vi "Check Packets.vi"(1 "A":string, 2 "B":string) -> (0 "A < B?":bool)   [LabVIEW 2022 SP3, in "AoC22.lvlib"]
uses:
  AoC22.lvlib
  Packet Parser.ctl
  Packet Token.ctl
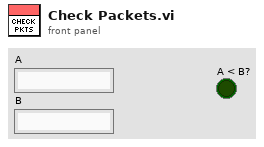
[diagram p1: front panel]
types:
  T1 = typedef "AoC22.lvlib/Packet Parser.ctl" = cluster{"String":string, "Next":i32}
  T2 = typedef "AoC22.lvlib/Packet Token.ctl" = enum16{"List", "End List", "Value", "Comma"}
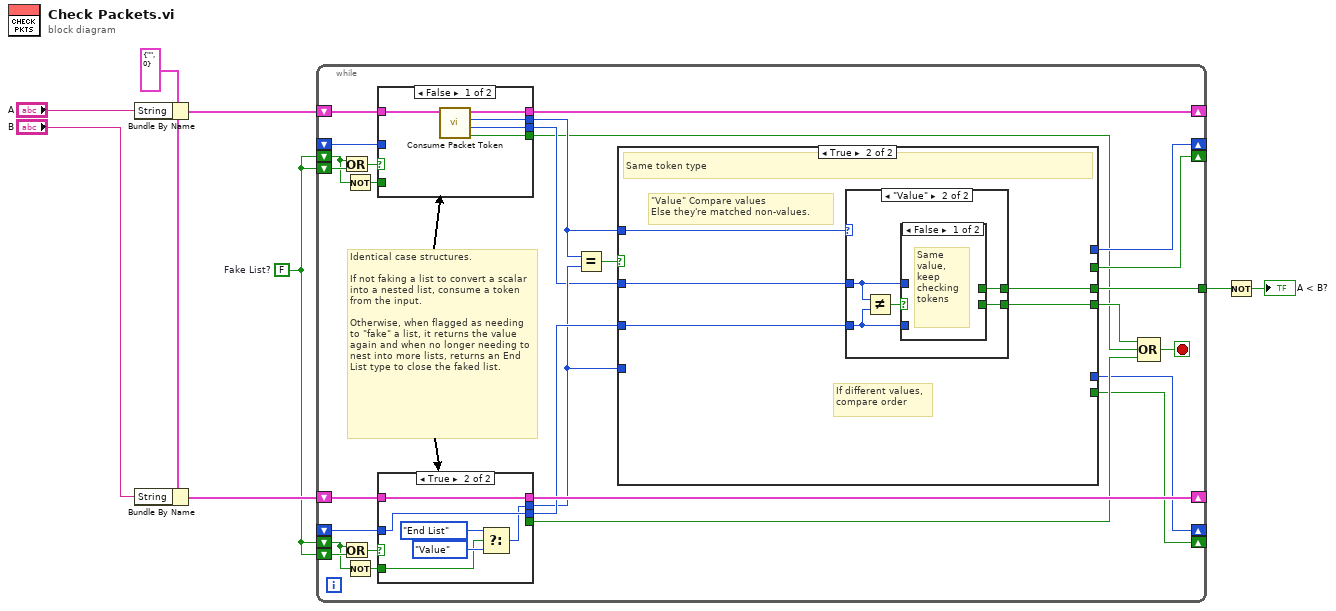
[diagram p0: block diagram]
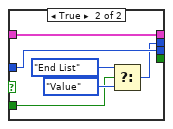
[diagram p2: hidden frame]
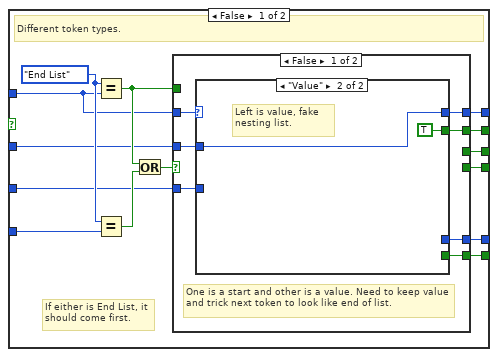
[diagram p3: hidden frame]
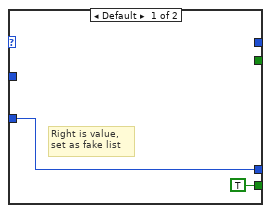
[diagram p4: hidden frame]
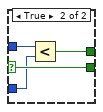
[diagram p7: hidden frame]
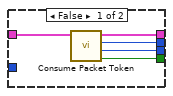
[diagram p8: hidden frame]
diagram:
  w5 = FALSE  # Fake List?
  w8 = T1 {"String"="", "Next"=0} ("Packet Parser")
  n1 = Bundle By Name(cluster=w8, "String"="A") -> (w7:T1)
  n2 = Bundle By Name(cluster=w8, "String"="B") -> (w6:T1)
  n3 = while {
    shift-right: [w16] -> _
    shift-left: w7 -> [w20]
    shift-right: [w34] -> _
    shift-left: w6 -> [w36]
    shift-right: [w25] -> _
    shift-left: w5 -> [w9]
    shift-right: [w24] -> _
    shift-left: w5 -> [w10]
    shift-right: [w26] -> _
    shift-left: _ -> [w19]
    shift-right: [w23] -> _
    shift-left: _ -> [w35]
    tunnel: [w28] -> w4
    shift-left: w5 -> [w17]
    shift-left: w5 -> [w21]
    stop <- w32 stop-if-true
    # "Identical case structures.\n\nIf not faking a list to convert a scalar into a nested list, consume a token from the input.\n\nOtherwise, when flagged as needing to \"fake\" a list, it returns the value again and when no longer needing to nest into more lists, returns an End List type to close the faked list."
    n4 = Or(x=w9, y=w17) -> (x .or. y?=w18:bool)
    n5 = Or(x=w10, y=w21) -> (x .or. y?=w22:bool)
    n6 = Not(x=w9) -> (.not. x?=w12:bool)
    n7 = Not(x=w10) -> (.not. x?=w11:bool)
    n8 = case shown="False" w18 {
      tunnel: w20 -> [w41 w47]
      tunnel: [w40 w47] -> w16
      tunnel: [w39 _] -> w13
      tunnel: [w38 w46] -> w14
      tunnel: [w37 w42] -> w15
      tunnel: w19 -> [_ w46]
      tunnel: w12 -> [_ w43]
      frame False {
        n9 = call "Consume Packet Token.vi"("Packet Parser In"=w41) -> ("End?"=w39:bool, "Value"=w38:i32, "Type"=w37:T2, "Packet Parser"=w40:T1)  [unwired: 7 in]
      }
      frame True {
        n10 = Select(t=Packet_Token."End List" ("Packet Token"), s=w43, f=Packet_Token."Value" ("Packet Token")) -> (s? t:f=w42:T2)
      }
    }
    n11 = case shown="True" w22 {
      tunnel: w36 -> [w93 w99]
      tunnel: [w92 w99] -> w34
      tunnel: [w91 _] -> w33
      tunnel: [w90 w98] -> w30
      tunnel: [w89 w94] -> w27
      tunnel: w35 -> [_ w98]
      tunnel: w11 -> [_ w95]
      frame False {
        n12 = call "Consume Packet Token.vi"("Packet Parser In"=w93) -> ("End?"=w91:bool, "Value"=w90:i32, "Type"=w89:T2, "Packet Parser"=w92:T1)  [unwired: 7 in]
      }
      frame True {
        n13 = Select(t=Packet_Token."End List" ("Packet Token"), s=w95, f=Packet_Token."Value" ("Packet Token")) -> (s? t:f=w94:T2)
      }
    }
    n14 = Equal?(x=w15, y=w27) -> (x = y?=w31:bool)
    n15 = case shown="True" w31 {
      tunnel: w15 -> [w52 w79]
      tunnel: w14 -> [w55 w78]
      tunnel: w30 -> [w54 w77]
      tunnel: [w56 w76] -> w29
      tunnel: [w57 w75] -> w28
      tunnel: w27 -> [w61 _]
      tunnel: [w51 _] -> w26
      tunnel: [w50 _] -> w25
      tunnel: [w49 _] -> w24
      tunnel: [w48 _] -> w23
      frame False {
        w60 = Packet_Token."End List" ("x")
        # "If either is End List, it should come first."
        # "Different token types."
        n16 = Equal?(x=w60, y=w52) -> (x = y?=w58:bool)
        n17 = Equal?(x=w60, y=w61) -> (x = y?=w59:bool)
        n18 = Or(x=w58, y=w59) -> (x .or. y?=w53:bool)
        n19 = case shown="False" w53 {
          selector: w53 -> [_ w73]
          tunnel: w58 -> [_ w74]
          tunnel: [_ w74] -> w57
          tunnel: [_ w73] -> w56
          tunnel: w55 -> [w67 _]
          tunnel: w54 -> [w64 _]
          tunnel: w52 -> [w68 _]
          tunnel: [w66 _] -> w51
          tunnel: [w65 _] -> w50
          tunnel: [w63 _] -> w49
          tunnel: [w62 _] -> w48
          frame False {
            # "One is a start and other is a value. Need to keep value and trick next token to look like end of list."
            n20 = case shown="\"Value\"" w68 {
              tunnel: w67 -> [_ w72]
              tunnel: [_ w72] -> w66
              tunnel: [_ TRUE] -> w65
              tunnel: w64 -> [w69 _]
              tunnel: [TRUE _] -> w63
              tunnel: [w69 _] -> w62
              frame Default {
                # "Right is value, set as fake list"
              }
              frame "Value" {
                # "Left is value, fake nesting list."
              }
            }
          }
          frame True {
            # "One is an end list and that one should come first."
          }
        }
      }
      frame True {
        # "\"Value\" Compare values\nElse they're matched non-values."
        # "If different values, compare order"
        # "Same token type"
        n21 = case shown="\"Value\"" w79 {
          tunnel: w78 -> [_ w83]
          tunnel: w77 -> [_ w82]
          tunnel: [_ w81] -> w76
          tunnel: [_ w80] -> w75
          frame Default {
            # "Matched non-value symbol."
          }
          frame "Value" {
            n22 = Not Equal?(x=w83, y=w82) -> (x != y?=w84:bool)
            n23 = case shown="False" w84 {
              selector: w84 -> [_ w88]
              tunnel: w83 -> [_ w87]
              tunnel: w82 -> [_ w86]
              tunnel: [_ w88] -> w81
              tunnel: [_ w85] -> w80
              frame False {
                # "Same value, keep checking tokens"
              }
              frame True {
                n24 = Less?(x=w87, y=w86) -> (x < y?=w85:bool)
              }
            }
          }
        }
      }
    }
    n25 = Compound Arithmetic op=OR(w29, w13, w33) -> (w32:bool)
  }
  n26 = Not(x=w4) -> (.not. x?=→"A < B?":bool)
